vi "Rubik Cube Solver Main.vi"() -> ()   [LabVIEW 2011]
uses:
  Typedef/cube.ctl
  Typedef/face.ctl
  Typedef/main state.ctl
  Typedef/colours.ctl
  Typedef/operation.ctl
panel:
  in  "show":bool
  in  "random seed":dbl=1234.0
  out "bottom corners solved?":bool
  out "bottom corners positioned?":bool
  out "bottom cross aligned?":bool
  out "bottom cross solved?":bool
  out "middle layer edges solved?":bool
  out "upper corners solved?":bool
  out "upper cross solved?":bool
  in  "start colour":T1
  in  "solve!":bool
  in  "rot up":bool
  in  "rot left":bool
  in  "rot right":bool
  in  "rot down":bool
  in  "unrandomise":bool
  out "operations":T2[](array[typedef])
  out "element":T2
  in  "rot L +":bool
  in  "rot B -":bool
  in  "rot B +":bool
  in  "rot R -":bool
  in  "rot R +":bool
  in  "rot L -":bool
  in  "iterations":i32=5000
  in  "randomise":bool
  in  "reset":bool
  in  "rot T -":bool
  in  "rot T +":bool
  in  "rot F -":bool
  in  "rot F +":bool
  out "cube":T3
  in  "stop":bool
  # "top edge"
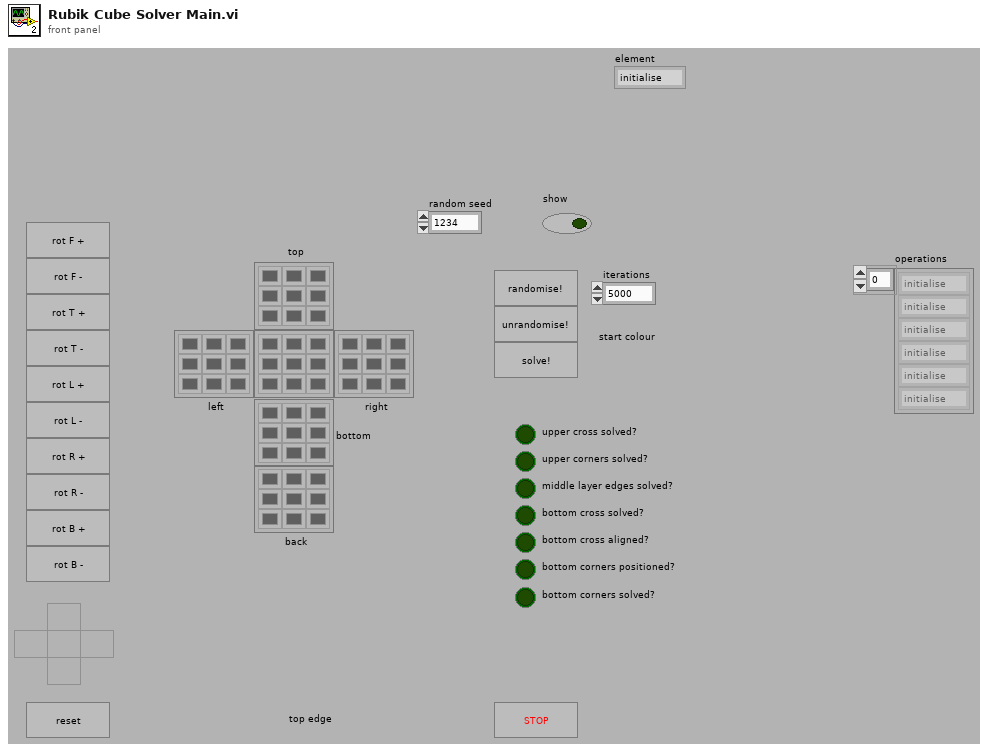
[diagram p1: front panel]
types:
  T1 = typedef "colours.ctl" = u16
  T2 = typedef "main state.ctl" = enum16{"initialise", "exit", "passthrough", "rotate F +", "rotate F -", "rotate T +", "rotate T -", "rotate L +", "rotate L -", "rotate R +", "rotate R -", "rotate B +", "rotate B -", "rotate up", "rotate left", "rotate right", "rotate down", "randomise", "unrandomise", "solve!", "solve step 1", "solve step 2", "solve step 3", "solve step 4", "solve step 5", "solve step 6", "solve step 7"}
  T3 = typedef "cube.ctl" = cluster{"top":T4, "left":T4, "right":T4, "bottom":T4, "back":T4, "front":T4}
  T4 = typedef "face.ctl" = u32[][]
  T5 = typedef "operation.ctl" = enum16{"nop", "T+", "T-", "F+", "F-", "L+", "L-", "R+", "R-", "B+", "B-", "<--", "-->", "^", "V"}
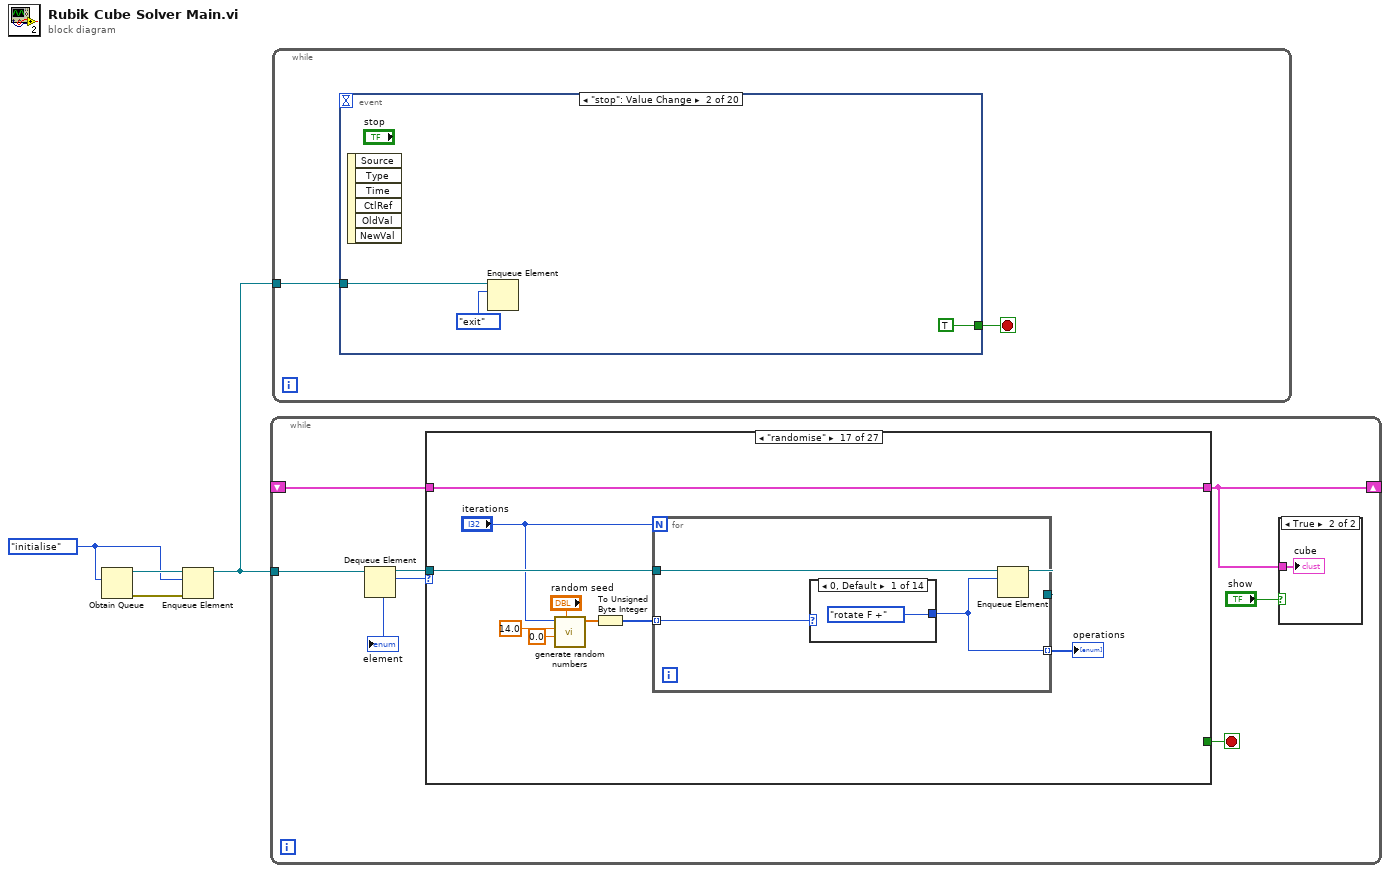
[diagram p0: block diagram]
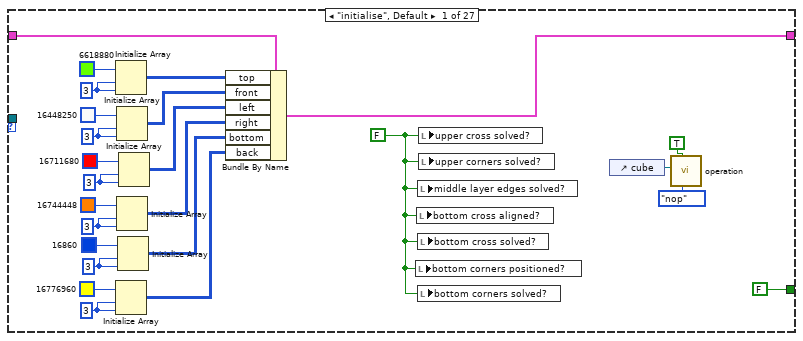
[diagram p3: hidden frame]
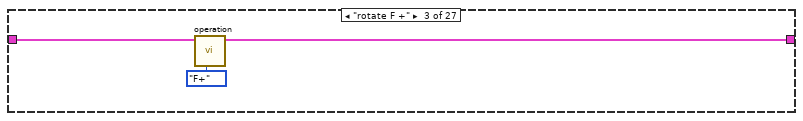
[diagram p5: hidden frame]
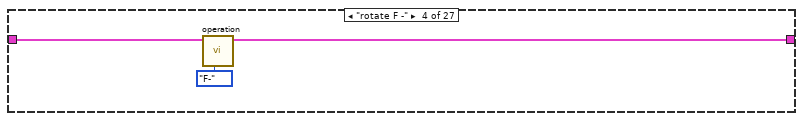
[diagram p6: hidden frame]
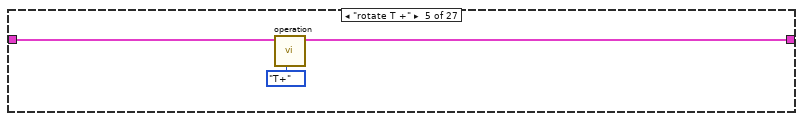
[diagram p7: hidden frame]
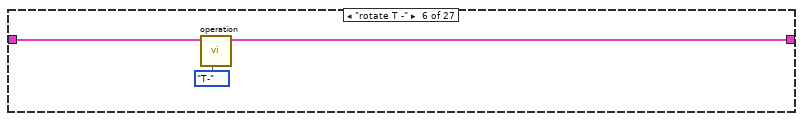
[diagram p8: hidden frame]
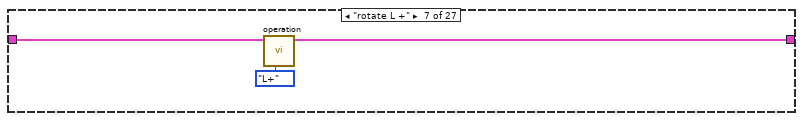
[diagram p9: hidden frame]
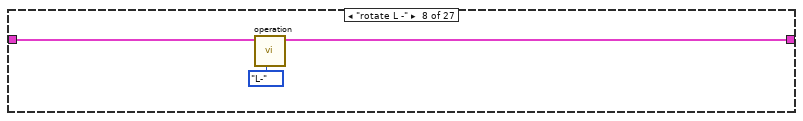
[diagram p10: hidden frame]
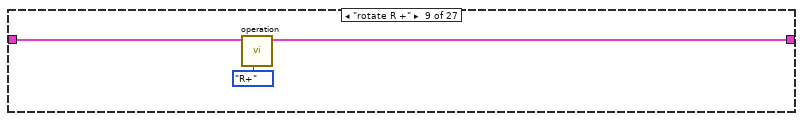
[diagram p11: hidden frame]
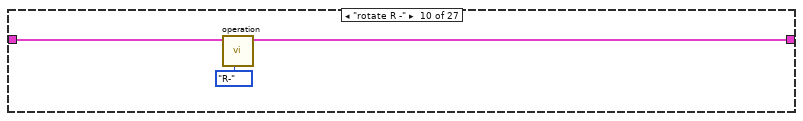
[diagram p12: hidden frame]
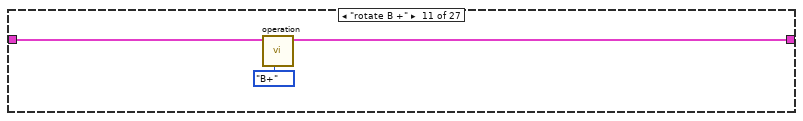
[diagram p13: hidden frame]
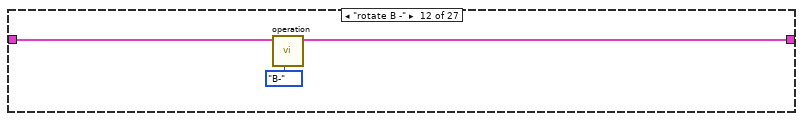
[diagram p14: hidden frame]
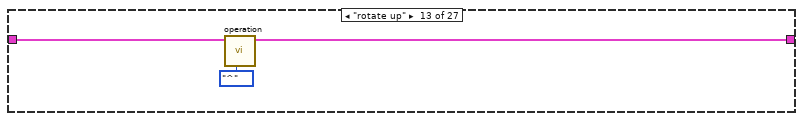
[diagram p15: hidden frame]
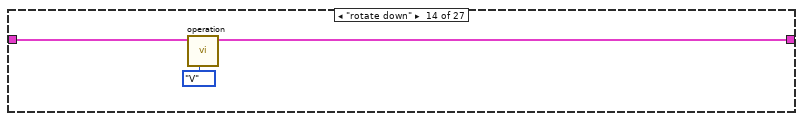
[diagram p16: hidden frame]
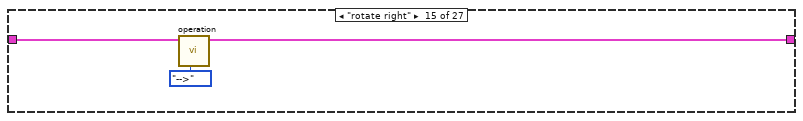
[diagram p17: hidden frame]
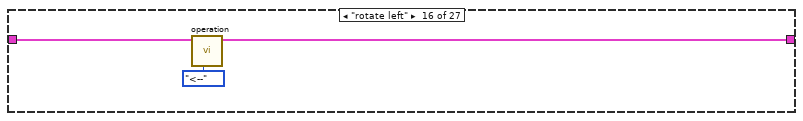
[diagram p18: hidden frame]
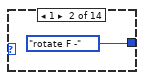
[diagram p19: hidden frame]
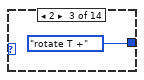
[diagram p20: hidden frame]
diagram:
  w2 = main_state."initialise" ("state")
  n1 = Obtain Queue(element data type=w2) -> (queue out=w4:refnum<queue>, error out=w3:errorcluster)  [unwired: 4 in, 1 out]
  n2 = Enqueue Element(queue=w4, element=w2, error in (no error)=w3) -> (queue out=w1:refnum<queue>)  [unwired: 1 in, 2 out]
  n3 = while {
    tunnel: w1 -> [w11]
    shift-right: [w9] -> _
    shift-left: _ -> [w8]
    stop <- w10 stop-if-true
    n4 = Dequeue Element(queue=w11) -> (queue out=w7:refnum<queue>, element=w6:T2)  [unwired: 2 in, 2 out]
    "element" <- w6
    n5 = case shown="\"randomise\"" w6 {
      tunnel: [FALSE _ _ _ _ _ _ _ _ _ _ _ _ _ _ _ _ _ _ _ _ _ _ _ _ _ TRUE] -> w10
      tunnel: w8 -> [w36 w38 w40 w43 w46 w49 w52 w55 w58 w61 w64 w67 w70 w73 w76 w79 w88 w108 w131 w138 w148 w151 w154 w158 w161 w164 w165]
      tunnel: [w17 w38 w39 w42 w45 w48 w51 w54 w57 w60 w63 w66 w69 w72 w75 w78 w88 w108 w131 w135 w145 w150 w153 w156 w160 w163 w165] -> w9
      tunnel: w7 -> [_ _ _ _ _ _ _ _ _ _ _ _ _ _ _ _ w89 w111 w132 _ _ _ _ _ _ _ _]
      frame "initialise", Default {
        w16 = FALSE ("upper cross solved?")
        w23 = 3 ("dimension size")
        w20 = 3 ("dimension size")
        w25 = 3 ("dimension size")
        w29 = 3 ("dimension size")
        w31 = 3 ("dimension size")
        w35 = 3 ("dimension size")
        n6 = Initialize Array(u32 6618880, w35, w35) -> (w33:u32[][])
        n7 = Initialize Array(u32 16776960, w23, w23) -> (w18:u32[][])
        n8 = Initialize Array(u32 16448250, w31, w31) -> (w30:u32[][])
        n9 = Initialize Array(u32 16744448, w25, w25) -> (w24:u32[][])
        n10 = Initialize Array(u32 16860, w20, w20) -> (w19:u32[][])
        n11 = Initialize Array(u32 16711680, w29, w29) -> (w27:u32[][])
        n12 = Bundle By Name(cluster=w36, "top"=w33, "front"=w30, "left"=w27, "right"=w24, "bottom"=w19, "back"=w18) -> (w17:T3)
        n13 = local write "bottom corners positioned?"(w16) -> ()
        n14 = local write "bottom cross aligned?"(w16) -> ()
        n15 = local write "middle layer edges solved?"(w16) -> ()
        n16 = local write "bottom cross solved?"(w16) -> ()
        n17 = local write "bottom corners solved?"(w16) -> ()
        n18 = local write "upper cross solved?"(w16) -> ()
        n19 = local write "upper corners solved?"(w16) -> ()
        n20 = control-ref of="cube"() -> (w13:refnum<vi>)
        n21 = call "operation.vi"("operation"=operation."nop", "clear buffer (F)"=TRUE, "cube"=w13) -> ()  [unwired: 7 in, 2 out]
      }
      frame "passthrough" {
      }
      frame "rotate F +" {
        n22 = call "operation.vi"("operation"=operation."F+", "cube in"=w40) -> ("cube out"=w39:T3)  [unwired: 8 in, 1 out]
      }
      frame "rotate F -" {
        n23 = call "operation.vi"("operation"=operation."F-", "cube in"=w43) -> ("cube out"=w42:T3)  [unwired: 8 in, 1 out]
      }
      frame "rotate T +" {
        n24 = call "operation.vi"("operation"=operation."T+", "cube in"=w46) -> ("cube out"=w45:T3)  [unwired: 8 in, 1 out]
      }
      frame "rotate T -" {
        n25 = call "operation.vi"("operation"=operation."T-", "cube in"=w49) -> ("cube out"=w48:T3)  [unwired: 8 in, 1 out]
      }
      frame "rotate L +" {
        n26 = call "operation.vi"("operation"=operation."L+", "cube in"=w52) -> ("cube out"=w51:T3)  [unwired: 8 in, 1 out]
      }
      frame "rotate L -" {
        n27 = call "operation.vi"("operation"=operation."L-", "cube in"=w55) -> ("cube out"=w54:T3)  [unwired: 8 in, 1 out]
      }
      frame "rotate R +" {
        n28 = call "operation.vi"("operation"=operation."R+", "cube in"=w58) -> ("cube out"=w57:T3)  [unwired: 8 in, 1 out]
      }
      frame "rotate R -" {
        n29 = call "operation.vi"("operation"=operation."R-", "cube in"=w61) -> ("cube out"=w60:T3)  [unwired: 8 in, 1 out]
      }
      frame "rotate B +" {
        n30 = call "operation.vi"("operation"=operation."B+", "cube in"=w64) -> ("cube out"=w63:T3)  [unwired: 8 in, 1 out]
      }
      frame "rotate B -" {
        n31 = call "operation.vi"("operation"=operation."B-", "cube in"=w67) -> ("cube out"=w66:T3)  [unwired: 8 in, 1 out]
      }
      frame "rotate up" {
        n32 = call "operation.vi"("operation"=operation."^", "cube in"=w70) -> ("cube out"=w69:T3)  [unwired: 8 in, 1 out]
      }
      frame "rotate down" {
        n33 = call "operation.vi"("operation"=operation."V", "cube in"=w73) -> ("cube out"=w72:T3)  [unwired: 8 in, 1 out]
      }
      frame "rotate right" {
        n34 = call "operation.vi"("operation"=operation."-->", "cube in"=w76) -> ("cube out"=w75:T3)  [unwired: 8 in, 1 out]
      }
      frame "rotate left" {
        n35 = call "operation.vi"("operation"=operation."<--", "cube in"=w79) -> ("cube out"=w78:T3)  [unwired: 8 in, 1 out]
      }
      frame "randomise" {
        n36 = call "generate random numbers.vi"("random seed"="random seed", "lowlim"=0.0, "highlim"=14.0, "number of elements"="iterations") -> ("random numbers"=w86:dbl[])  [unwired: 6 in, 1 out]
        n37 = To Unsigned Byte Integer(number=w86) -> (unsigned 8bit integer=w85:u8[])
        n38 = for {
          N: "iterations" -> [_]
          tunnel: w89 -> [w93]
          tunnel: [w92] -> w87 mode=indexing
          tunnel: w85 -> [w91] mode=indexing
          tunnel: [w90] -> _
          n39 = case shown="0, Default" w91 {
            tunnel: [main_state."rotate F +" ("state") main_state."rotate F -" ("state") main_state."rotate T +" ("state") main_state."rotate T -" ("state") main_state."rotate L +" ("state") main_state."rotate L -" ("state") main_state."rotate R +" ("state") main_state."rotate R -" ("state") main_state."rotate B +" ("state") main_state."rotate B -" ("state") main_state."rotate up" ("state") main_state."rotate left" ("state") main_state."rotate right" ("state") main_state."rotate down" ("state")] -> w92
            frame 0, Default {
            }
            frame 1 {
            }
            frame 2 {
            }
            frame 3 {
            }
            frame 4 {
            }
            frame 5 {
            }
            frame 6 {
            }
            frame 7 {
            }
            frame 8 {
            }
            frame 9 {
            }
            frame 10 {
            }
            frame 11 {
            }
            frame 12 {
            }
            frame 13 {
            }
          }
          n40 = Enqueue Element(queue=w93, element=w92) -> (queue out=w90:refnum<queue>)  [unwired: 2 in, 2 out]
        }
        "operations" <- w87
      }
      frame "unrandomise" {
        n41 = local read "operations"() -> (w110:T2[])
        n42 = Reverse 1D Array(array=w110) -> (reversed array=w109:T2[])
        n43 = for {
          tunnel: w109 -> [w113] mode=indexing
          tunnel: w111 -> [w114]
          n44 = case shown="Default" w113 {
            tunnel: [main_state."rotate F -" ("element") main_state."rotate F +" ("element") main_state."rotate T -" ("element") main_state."rotate T +" ("element") main_state."rotate L -" ("element") main_state."rotate L +" ("element") main_state."rotate R -" ("element") main_state."rotate R +" ("element") main_state."rotate B -" ("element") main_state."rotate B +" ("element") main_state."rotate down" ("element") main_state."rotate right" ("element") main_state."rotate left" ("element") main_state."rotate up" ("element") main_state."passthrough" ("element")] -> w112
            frame "rotate F +" {
            }
            frame "rotate F -" {
            }
            frame "rotate T +" {
            }
            frame "rotate T -" {
            }
            frame "rotate L +" {
            }
            frame "rotate L -" {
            }
            frame "rotate R +" {
            }
            frame "rotate R -" {
            }
            frame "rotate B +" {
            }
            frame "rotate B -" {
            }
            frame "rotate up" {
            }
            frame "rotate left" {
            }
            frame "rotate right" {
            }
            frame "rotate down" {
            }
            frame Default {
            }
          }
          n45 = Enqueue Element(queue=w114, element=w112) -> ()  [unwired: 2 in, 3 out]
        }
      }
      frame "solve!" {
        w130 = T2[] [enum."solve step 1", enum."solve step 2", enum."solve step 3", enum."solve step 4", enum."solve step 5", enum."solve step 6", enum."solve step 7"] items=["initialise", "exit", "passthrough", "rotate F +", "rotate F -", "rotate T +", "rotate T -", "rotate L +", "rotate L -", "rotate R +", "rotate R -", "rotate B +", "rotate B -", "rotate up", "rotate left", "rotate right", "rotate down", "randomise", "unrandomise", "solve!", "solve step 1", "solve step 2", "solve step 3", "solve step 4", "solve step 5", "solve step 6", "solve step 7"]
        n46 = for {
          tunnel: w132 -> [w134]
          tunnel: w130 -> [w133] mode=indexing
          n47 = Enqueue Element(queue=w134, element=w133) -> ()  [unwired: 2 in, 3 out]
        }
      }
      frame "solve step 1" {
        n48 = Index Array(array=u32[] [16711680, 16860, 6618880, 16776960, 16448250, 16744448], index="start colour") -> (element=w139:u32)
        n49 = call "step1_FindStartPiece.vi"("start colour"=w139, "cube in"=w138) -> ("cube out"=w136:T3)  [unwired: 8 in, 1 out]
        n50 = call "step1 SolveUpperCross.vi"("cube in"=w136) -> ("upper cross solved?"=→"upper cross solved?":bool, "cube out"=w135:T3)  [unwired: 8 in, 1 out]
      }
      frame "solve step 2" {
        n51 = call "step2 Solve.vi"("cube in"=w148) -> ("upper layer solved?"=→"upper corners solved?":bool, "cube out"=w146:T3)  [unwired: 8 in, 1 out]
        n52 = call "operation.vi"("operation"=operation."V", "cube in"=w146) -> ("cube out"=w142:T3)  [unwired: 8 in, 1 out]
        n53 = call "operation.vi"("operation"=operation."V", "cube in"=w142) -> ("cube out"=w145:T3)  [unwired: 8 in, 1 out]
      }
      frame "solve step 3" {
        n54 = call "step3 Solve.vi"("cube in"=w151) -> ("middle layer solved?"=→"middle layer edges solved?":bool, "cube out"=w150:T3)  [unwired: 8 in, 1 out]
      }
      frame "solve step 4" {
        n55 = call "step4 Solve.vi"("cube in"=w154) -> ("upper cross solved?"=→"bottom cross solved?":bool, "cube out"=w153:T3)  [unwired: 8 in, 1 out]
      }
      frame "solve step 5" {
        n56 = call "step5 AlignFrontEdge.vi"("cube in"=w158) -> ("cube out"=w157:T3)  [unwired: 9 in, 1 out]
        n57 = call "step5 TestAndAlignUpperCross.vi"("cube in"=w157) -> ("cube out"=w156:T3)  [unwired: 10 in]
        n58 = call "step5 TestIfUpperCrossAligned.vi"("cube in"=w156) -> ("upper cross aligned?"=→"bottom cross aligned?":bool)  [unwired: 9 in, 1 out]
      }
      frame "solve step 6" {
        n59 = call "step6 Solve.vi"("cube in"=w161) -> ("all corners solved?"=→"bottom corners positioned?":bool, "cube out"=w160:T3)  [unwired: 8 in, 1 out]
      }
      frame "solve step 7" {
        n60 = call "step7 Solve.vi"("cube in"=w164) -> ("all corners solved?"=→"bottom corners solved?":bool, "cube out"=w163:T3)  [unwired: 9 in]
      }
      frame "exit" {
      }
    }
    n61 = case shown="True" "show" {
      tunnel: w9 -> [_ w12]
      frame False {
      }
      frame True {
        "cube" <- w12
      }
    }
  }
  n62 = while {
    tunnel: w1 -> [w168]
    stop <- w167 stop-if-true
    n63 = event shown="[1] \"stop\": Value Change" {
      selector: _ -> [_ _ _ _ _ _ _ _ _ _ _ _ _ _ _ _ _ _ _ _]
      dyn-events: _ -> [_ _ _ _ _ _ _ _ _ _ _ _ _ _ _ _ _ _ _ _]
      timeout: _ -> [_ _ _ _ _ _ _ _ _ _ _ _ _ _ _ _ _ _ _ _]
      tunnel: w168 -> [_ w171 w174 w177 w180 w183 w184 w187 w189 w191 w193 w195 w197 w201 w204 w207 w210 w213 w216 w219]
      tunnel: [_ TRUE FALSE FALSE FALSE FALSE _ _ _ _ _ _ _ FALSE FALSE FALSE FALSE FALSE FALSE FALSE] -> w167
      event Timeout {
        n64 = event-data() -> ()  [unwired: 1 in, 2 out]
      }
      event "stop": Value Change {
        n65 = event-data() -> ()  [unwired: 1 in, 6 out]
        n66 = Enqueue Element(queue=w171, element=main_state."exit" ("state")) -> ()  [unwired: 2 in, 3 out]
      }
      event "rot F +": Value Change {
        n67 = event-data() -> ()  [unwired: 1 in, 6 out]
        n68 = Enqueue Element(queue=w174, element=main_state."rotate F +" ("state")) -> ()  [unwired: 2 in, 3 out]
      }
      event "rot F -": Value Change {
        n69 = event-data() -> ()  [unwired: 1 in, 6 out]
        n70 = Enqueue Element(queue=w177, element=main_state."rotate F -" ("state")) -> ()  [unwired: 2 in, 3 out]
      }
      event "rot T +": Value Change {
        n71 = event-data() -> ()  [unwired: 1 in, 6 out]
        n72 = Enqueue Element(queue=w180, element=main_state."rotate T +" ("state")) -> ()  [unwired: 2 in, 3 out]
      }
      event "rot T -": Value Change {
        n73 = event-data() -> ()  [unwired: 1 in, 6 out]
        n74 = Enqueue Element(queue=w183, element=main_state."rotate T -" ("state")) -> ()  [unwired: 2 in, 3 out]
      }
      event "rot L +": Value Change {
        n75 = event-data() -> ()  [unwired: 1 in, 6 out]
        n76 = Enqueue Element(queue=w184, element=main_state."rotate L +" ("state")) -> ()  [unwired: 2 in, 3 out]
      }
      event "solve!": Value Change {
        w186 = FALSE ("upper cross solved?")
        n77 = event-data() -> ()  [unwired: 1 in, 6 out]
        n78 = Enqueue Element(queue=w187, element=main_state."solve!" ("state")) -> ()  [unwired: 2 in, 3 out]
        n79 = local write "bottom corners positioned?"(w186) -> ()
        n80 = local write "bottom cross aligned?"(w186) -> ()
        n81 = local write "middle layer edges solved?"(w186) -> ()
        n82 = local write "bottom cross solved?"(w186) -> ()
        n83 = local write "bottom corners solved?"(w186) -> ()
        n84 = local write "upper cross solved?"(w186) -> ()
        n85 = local write "upper corners solved?"(w186) -> ()
      }
      event "rot L -": Value Change {
        n86 = event-data() -> ()  [unwired: 1 in, 6 out]
        n87 = Enqueue Element(queue=w189, element=main_state."rotate L -" ("state")) -> ()  [unwired: 2 in, 3 out]
      }
      event "rot R +": Value Change {
        n88 = event-data() -> ()  [unwired: 1 in, 6 out]
        n89 = Enqueue Element(queue=w191, element=main_state."rotate R +" ("state")) -> ()  [unwired: 2 in, 3 out]
      }
      event "rot R -": Value Change {
        n90 = event-data() -> ()  [unwired: 1 in, 6 out]
        n91 = Enqueue Element(queue=w193, element=main_state."rotate R -" ("state")) -> ()  [unwired: 2 in, 3 out]
      }
      event "rot B +": Value Change {
        n92 = event-data() -> ()  [unwired: 1 in, 6 out]
        n93 = Enqueue Element(queue=w195, element=main_state."rotate B +" ("state")) -> ()  [unwired: 2 in, 3 out]
      }
      event "rot B -": Value Change {
        n94 = event-data() -> ()  [unwired: 1 in, 6 out]
        n95 = Enqueue Element(queue=w197, element=main_state."rotate B -" ("state")) -> ()  [unwired: 2 in, 3 out]
      }
      event "rot up": Value Change {
        n96 = event-data() -> ()  [unwired: 1 in, 6 out]
        n97 = Enqueue Element(queue=w201, element=main_state."rotate up" ("state")) -> ()  [unwired: 2 in, 3 out]
      }
      event "rot left": Value Change {
        n98 = event-data() -> ()  [unwired: 1 in, 6 out]
        n99 = Enqueue Element(queue=w204, element=main_state."rotate left" ("state")) -> ()  [unwired: 2 in, 3 out]
      }
      event "rot right": Value Change {
        n100 = event-data() -> ()  [unwired: 1 in, 6 out]
        n101 = Enqueue Element(queue=w207, element=main_state."rotate right" ("state")) -> ()  [unwired: 2 in, 3 out]
      }
      event "rot down": Value Change {
        n102 = event-data() -> ()  [unwired: 1 in, 6 out]
        n103 = Enqueue Element(queue=w210, element=main_state."rotate down" ("state")) -> ()  [unwired: 2 in, 3 out]
      }
      event "reset": Value Change {
        n104 = event-data() -> ()  [unwired: 1 in, 6 out]
        n105 = Enqueue Element(queue=w213, element=main_state."initialise" ("state")) -> ()  [unwired: 2 in, 3 out]
      }
      event "randomise": Value Change {
        n106 = event-data() -> ()  [unwired: 1 in, 6 out]
        n107 = Enqueue Element(queue=w216, element=main_state."randomise" ("state")) -> ()  [unwired: 2 in, 3 out]
      }
      event "unrandomise": Value Change {
        n108 = event-data() -> ()  [unwired: 1 in, 6 out]
        n109 = Enqueue Element(queue=w219, element=main_state."unrandomise" ("state")) -> ()  [unwired: 2 in, 3 out]
      }
    }
  }
